vi "SetParameter.vi"(8 "error in (no error)":errorcluster, 10 "SetParameter":T1, 11 "AcPwrBase in":refnum<class "AcPwrBase.lvclass">) -> (0 "error out":errorcluster, 2 "StatusUpdates":string[](array[string]), 3 "AcPwrBase out":refnum<class "AcPwrBase.lvclass">)   [LabVIEW 2018, in "AcPwrPlugins.lvlib" / "AcPwrBase.lvclass"]
uses:
  AcPwrBase.lvclass
  TypeDefs/SetParameterInputs.ctl
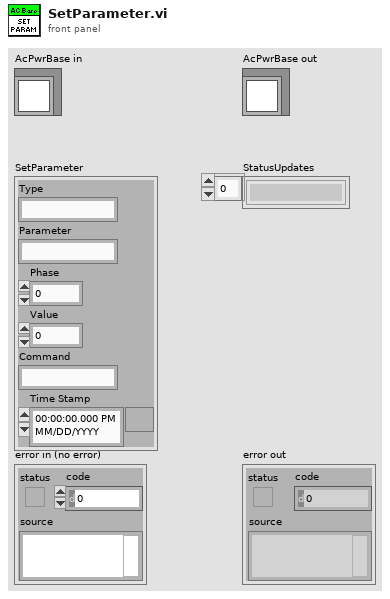
[diagram p1: front panel]
types:
  T1 = typedef "AcPwrPlugins.lvlib/AcPwrBase.lvclass/SetParameterInputs.ctl" = cluster{"Type":string, "Parameter":string, "Phase":i32, "Value":dbl, "Command":string, "Time Stamp":timestamp}
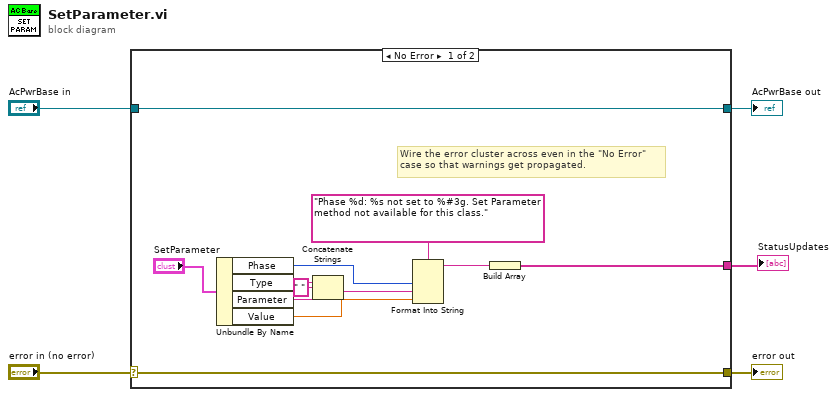
[diagram p0: block diagram]
diagram:
  n1 = case shown="No Error" "error in (no error)" {
    selector: "error in (no error)" -> [w16 w19]
    tunnel: [w16 w19] -> w4
    tunnel: [w17 w18] -> w2
    tunnel: "AcPwrBase in" -> [w17 w18]
    tunnel: [w6 _] -> w1
    frame No Error {
      # "Wire the error cluster across even in the \"No Error\"\ncase so that warnings get propagated."
      n2 = Unbundle By Name("SetParameter") -> ("Phase"=w12:i32, "Type"=w8:string, "Parameter"=w11:string, "Value"=w10:dbl)
      n3 = Concatenate Strings(w8, " " ("string"), w11) -> (w9:string)
      n4 = Format Into String(format string="Phase %d: %s not set to %#3g. Set Parameter method not available for this class.", w12, w9, w10) -> (resulting string=w14:string)  [unwired: 2 in, 1 out]
      n5 = Build Array(w14) -> (w6:string[])
    }
    frame Error {
    }
  }
  "error out" <- w4
  "AcPwrBase out" <- w2
  "StatusUpdates" <- w1
